vi "Find Flatten Terminals.vi"(8 "error in (no error)":errorcluster, 9 "BD":refnum<vi>, 11 "LV-Protoc in":refnum<class "LV-Protoc.lvclass">) -> (0 "error out":errorcluster, 2 "Output Term":refnum<vi>, 3 "LV-Protoc out":refnum<class "LV-Protoc.lvclass">)   [LabVIEW 2020, in "LV-Protoc.lvlib" / "LV-Protoc.lvclass"]
uses:
  LV-Protoc.lvclass
  <vilib>/Utility/traverseref.llb/TRef TravTarget.ctl
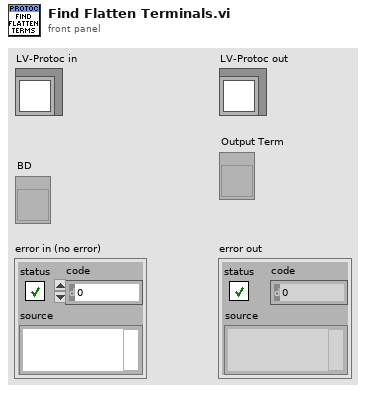
[diagram p1: front panel]
types:
  T1 = typedef "TRef TravTarget.ctl" = enum16{"FP", "BD", "Other"}
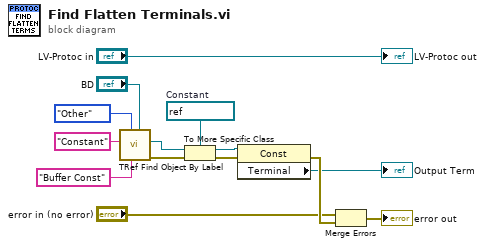
[diagram p0: block diagram]
diagram:
  w8 = refnum<vi> refnum  # Constant
  n1 = call <vilib>:"TRef Find Object By Label.vi"("Other Refnum"="BD", "Label"="Buffer Const", "Traverse Target"=TRef_TravTarget."Other", "Class Name"="Constant") -> ("error out"=w9:errorcluster, "Found Obj Ref"=w10:refnum<vi>)  [unwired: 4 in, 2 out]
  n2 = To More Specific Class(target class=w8, reference=w10, error in=w9) -> (specific class reference=w7:refnum<vi>, error out=w2:errorcluster)
  n3 = property class="Const"(reference=w7, error in=w2) -> (error out=w14:errorcluster, "Terminal"=→"Output Term":refnum<vi>)  [unwired: 1 out]
  n4 = Merge Errors("error in (no error)", w14) -> (→"error out":errorcluster)
  "LV-Protoc out" <- "LV-Protoc in"
